vi "DSF.Engine.Framework.Rx.vi"(8 "error in (no error)":errorcluster, 11 "Framework in":refnum<class "DSF.Engine.Framework.lvclass">) -> (0 "error out":errorcluster, 3 "Framework out":refnum<class "DSF.Engine.Framework.lvclass">)   [LabVIEW 2017, in "DSF.Engine.lvlib" / "DSF.Engine.Framework.lvclass"]
uses:
  DSF.Engine.Framework.lvclass
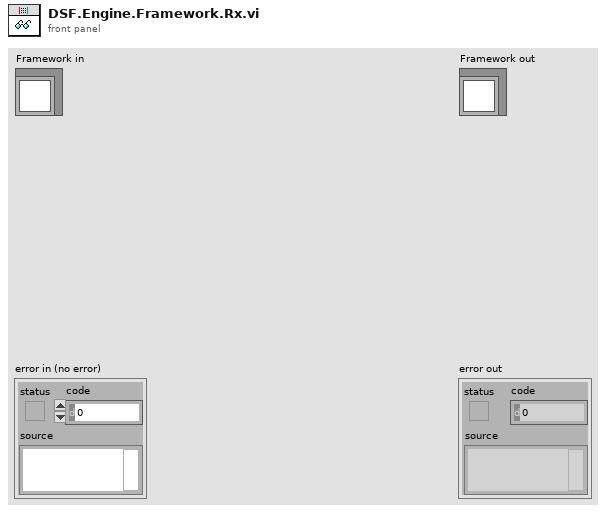
[diagram p1: front panel]
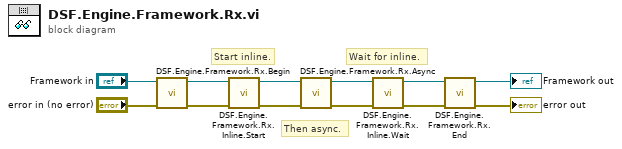
[diagram p0: block diagram]
diagram:
  # "Wait for inline."
  # "Start inline."
  # "Then async."
  n1 = call "DSF.Engine.Framework.Rx.Begin.vi"("error in (no error)"="error in (no error)", "Framework in"="Framework in") -> ("error out"=w9:errorcluster, "Framework out"=w10:refnum<class "DSF.Engine.Framework.lvclass">)  [unwired: 8 in]
  n2 = call "DSF.Engine.Framework.Rx.Inline.Start.vi"("error in (no error)"=w9, "Framework in"=w10) -> ("error out"=w1:errorcluster, "Framework out"=w2:refnum<class "DSF.Engine.Framework.lvclass">)  [unwired: 8 in]
  n3 = call "DSF.Engine.Framework.Rx.Async.vi"("error in (no error)"=w1, "Framework in"=w2) -> ("error out"=w4:errorcluster, "Framework out"=w3:refnum<class "DSF.Engine.Framework.lvclass">)  [unwired: 8 in]
  n4 = call "DSF.Engine.Framework.Rx.Inline.Wait.vi"("error in (no error)"=w4, "Framework in"=w3) -> ("error out"=w8:errorcluster, "Framework out"=w7:refnum<class "DSF.Engine.Framework.lvclass">)  [unwired: 8 in]
  n5 = call "DSF.Engine.Framework.Rx.End.vi"("error in (no error)"=w8, "Framework in"=w7) -> ("error out"=→"error out":errorcluster, "Framework out"=→"Framework out":refnum<class "DSF.Engine.Framework.lvclass">)  [unwired: 8 in]
